vi "Input_Commands_Flywheel.vi"(11 "All Joysticks":T1) -> (3 "Flywheel Commands":T4)   [LabVIEW 2012]
uses:
  Input_Commands_Flywheel.ctl
  Input_All_Joysticks.ctl
  Input_Single_Joystick.ctl
  <vilib>/Rock Robotics/WPI/Joystick/WPI_JoystickButtonState.ctl
panel:
  in  "Adjust Amount":dbl=5.0
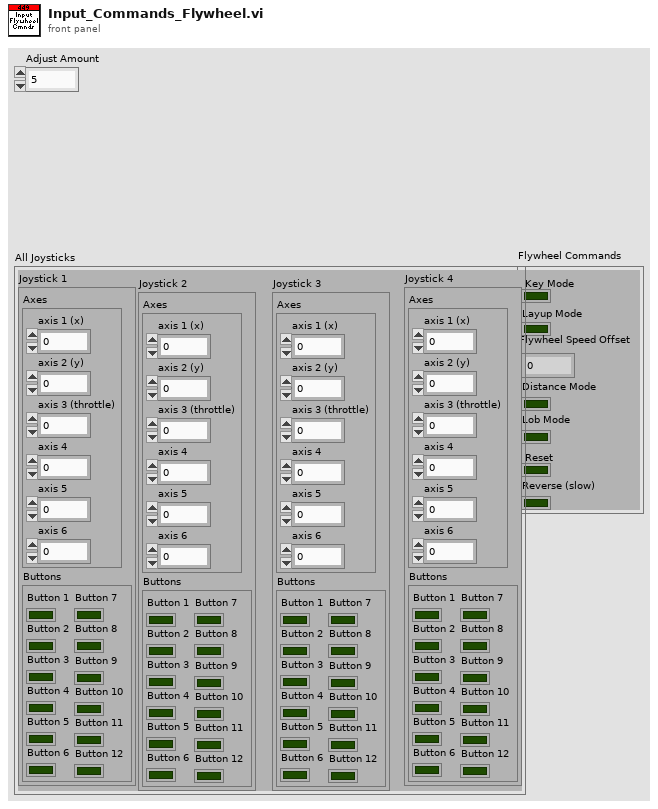
[diagram p1: front panel]
types:
  T1 = typedef "Input_All_Joysticks.ctl" = cluster{"Joystick 1":T2, "Joystick 2":T2, "Joystick 3":T2, "Joystick 4":T2}
  T2 = typedef "Input_Single_Joystick.ctl" = cluster{"Axes":cluster{"axis 1 (x)":dbl, "axis 2 (y)":dbl, "axis 3 (throttle)":dbl, "axis 4":dbl, "axis 5":dbl, "axis 6":dbl}, "Buttons":T3}
  T3 = typedef "WPI_JoystickButtonState.ctl" = cluster{"Button 1":bool, "Button 2":bool, "Button 3":bool, "Button 4":bool, "Button 5":bool, "Button 6":bool, "Button 7":bool, "Button 8":bool, "Button 9":bool, "Button 10":bool, "Button 11":bool, "Button 12":bool}
  T4 = typedef "Input_Commands_Flywheel.ctl" = cluster{"Key Mode":bool, "Layup Mode":bool, "Flywheel Speed Offset":dbl, "Distance Mode":bool, "Lob Mode":bool, "Reset":bool, "Reverse (slow)":bool}
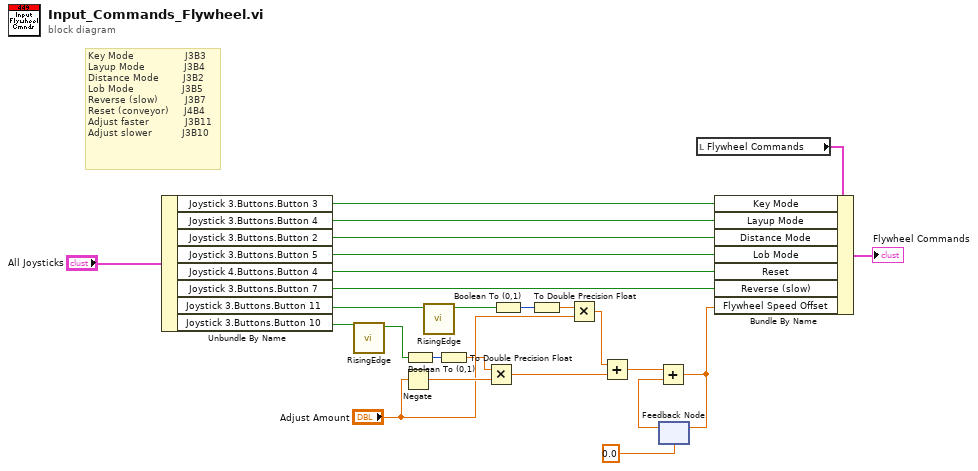
[diagram p0: block diagram]
diagram:
  # "Key Mode                 J3B3\nLayup Mode             J3B4\nDistance Mode        J3B2\nLob Mode                J3B5\nReverse (slow)         J3B7\nReset (conveyor)     J4B4\nAdjust faster            J3B11\nAdjust slower          J3B10"
  n1 = Unbundle By Name("All Joysticks") -> ("Joystick 3.Buttons.Button 3"=w22:bool, "Joystick 3.Buttons.Button 4"=w21:bool, "Joystick 3.Buttons.Button 2"=w20:bool, "Joystick 3.Buttons.Button 5"=w19:bool, "Joystick 4.Buttons.Button 4"=w18:bool, "Joystick 3.Buttons.Button 7"=w17:bool, "Joystick 3.Buttons.Button 11"=w14:bool, "Joystick 3.Buttons.Button 10"=w15:bool)
  n2 = call "RisingEdge.vi"("BooleanIn"=w15) -> ("BooleanOut"=w13:bool)  [unwired: 10 in]
  n3 = Negate(x="Adjust Amount") -> (-x=w10:dbl)
  n4 = Boolean To (0,1)(Boolean=w13) -> (0, 1=w11:i16)
  n5 = call "RisingEdge.vi"("BooleanIn"=w14) -> ("BooleanOut"=w12:bool)  [unwired: 10 in]
  n6 = To Double Precision Float(number=w11) -> (double precision float=w1:dbl)
  n7 = Multiply(x=w1, y=w10) -> (x*y=w6:dbl)
  n8 = Boolean To (0,1)(Boolean=w12) -> (0, 1=w9:i16)
  n9 = To Double Precision Float(number=w9) -> (double precision float=w2:dbl)
  n10 = Multiply(x=w2, y="Adjust Amount") -> (x*y=w7:dbl)
  n11 = Add(x=w7, y=w6) -> (x+y=w5:dbl)
  n12 = feedback #1(0.0) -> (w4:dbl)
  n13 = Add(x=w5, y=w4) -> (x+y=w3:dbl)
  n14 = feedback-in #1(w3) -> ()
  n15 = local read "Flywheel Commands"() -> (w24:T4)
  n16 = Bundle By Name(cluster=w24, "Key Mode"=w22, "Layup Mode"=w21, "Distance Mode"=w20, "Lob Mode"=w19, "Reset"=w18, "Reverse (slow)"=w17, "Flywheel Speed Offset"=w3) -> (→"Flywheel Commands":T4)
